vi "setROI.vi"(0 "PCO in":refnum<class "PCO_Camera.lvclass">, 7 "Seperator":string, 9 "value":string, 11 "error in (no error)":errorcluster) -> (4 "PCO out":refnum<class "PCO_Camera.lvclass">, 6 "output cluster":T1, 8 "value":dbl, 10 "Command out":string, 15 "error out":errorcluster)   [LabVIEW 2020, in "PCO_Camera.lvclass"]
uses:
  PCO_Camera.lvclass
  C:/GEECS/Developers Version/source/Device Drivers/Point Grey Camera/Point Grey Camera.lvclass
  ROI_TypDef.ctl
  PCO_Camera.lvclass/PCO_Camera.ctl
  Point Grey Camera.lvclass/Point Grey Camera.ctl
  Read Settings 2.vi
  Camera.lvclass
panel:
  out "ROI":u32[](array[numeric])
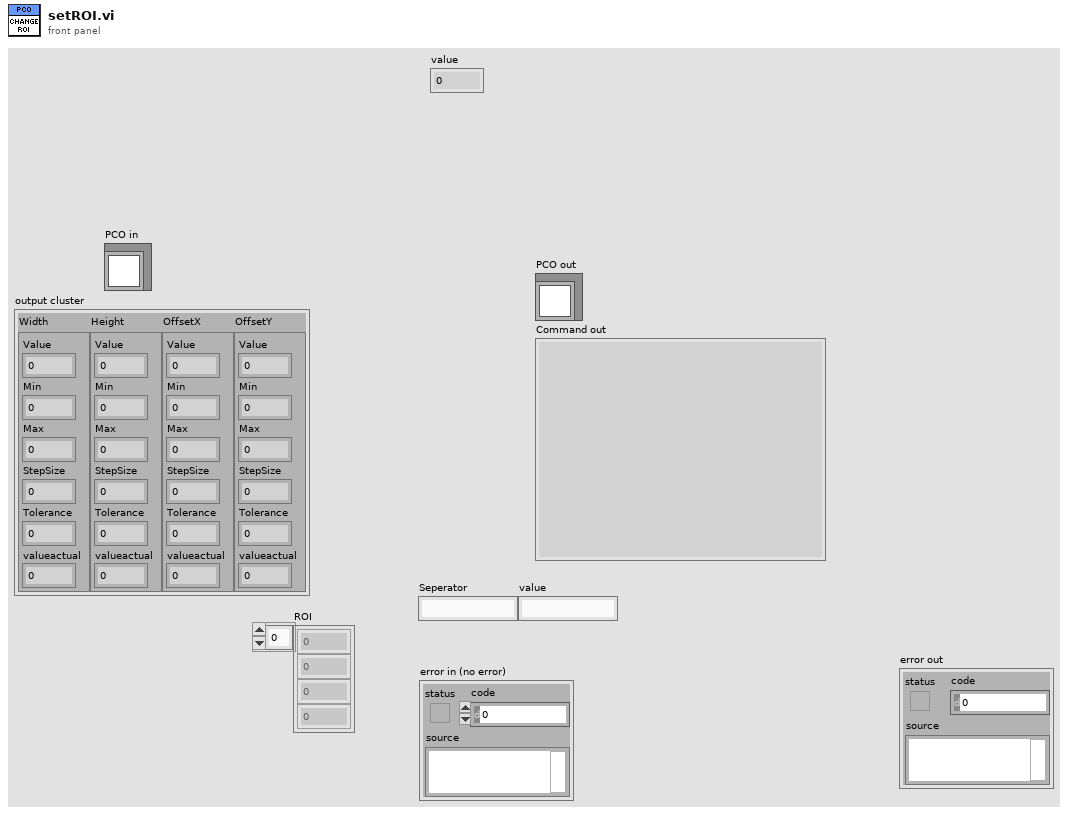
[diagram p1: front panel]
types:
  T1 = typedef "ROI_TypDef.ctl" = cluster{"Width":cluster{"Value":dbl, "Min":dbl, "Max":dbl, "StepSize":dbl, "Tolerance":dbl, "valueactual":dbl}, "Height":cluster{"Value":dbl, "Min":dbl, "Max":dbl, "StepSize":dbl, "Tolerance":dbl, "valueactual":dbl}, "OffsetX":cluster{"Value":dbl, "Min":dbl, "Max":dbl, "StepSize":dbl, "Tolerance":dbl, "valueactual":dbl}, "OffsetY":cluster{"Value":dbl, "Min":dbl, "Max":dbl, "StepSize":dbl, "Tolerance":dbl, "valueactual":dbl}}
  T2 = typedef "Point Grey Camera.lvclass/SettingsTypdef.ctl" = cluster{"Trigger":T3, "Gain":cluster{"Value":dbl, "Min":dbl, "Max":dbl, "StepSize":dbl, "Tolerance":dbl, "valueactual":dbl}, "Exposure":cluster{"Value":dbl, "Min":dbl, "Max":dbl, "StepSize":dbl, "Tolerance":dbl, "valueactual":dbl}, "Timeout":cluster{"Value":dbl, "Min":dbl, "Max":dbl, "StepSize":dbl, "Tolerance":dbl, "valueactual":dbl}, "LocalSavingPath":path, "Save":T3, "TriggerDelay":cluster{"Value":dbl, "Min":dbl, "Max":dbl, "StepSize":dbl, "Tolerance":dbl, "valueactual":dbl}, "CamSession":string, "ROI":T1, "MaxGUIPixel":cluster{"Value":dbl, "Min":dbl, "Max":dbl, "StepSize":dbl, "Tolerance":dbl, "valueactual":dbl}, "Target":cluster{"X":cluster{"Value":dbl, "Min":dbl, "Max":dbl, "StepSize":dbl, "Tolerance":dbl, "valueactual":dbl}, "Y":cluster{"Value":dbl, "Min":dbl, "Max":dbl, "StepSize":dbl, "Tolerance":dbl, "valueactual":dbl}}, "Analysis":T3, "maxshot#":dbl, "SpatialCalibration":cluster{"Value":dbl, "Min":dbl, "Max":dbl, "StepSize":dbl, "Tolerance":dbl, "valueactual":dbl}, "roistatus":T3, "Lineout":T3, "AnalysisThreshold":cluster{"Value":dbl, "Min":dbl, "Max":dbl, "StepSize":dbl, "Tolerance":dbl, "valueactual":dbl}, "TargetSize":cluster{"X":cluster{"Value":dbl, "Min":dbl, "Max":dbl, "StepSize":dbl, "Tolerance":dbl, "valueactual":dbl}, "Y":cluster{"Value":dbl, "Min":dbl, "Max":dbl, "StepSize":dbl, "Tolerance":dbl, "valueactual":dbl}}, "Simulation":T3, "SpatialCalibrationY":cluster{"Value":dbl, "Min":dbl, "Max":dbl, "StepSize":dbl, "Tolerance":dbl, "valueactual":dbl}, "Target2":cluster{"X":cluster{"Value":dbl, "Min":dbl, "Max":dbl, "StepSize":dbl, "Tolerance":dbl, "valueactual":dbl}, "Y":cluster{"Value":dbl, "Min":dbl, "Max":dbl, "StepSize":dbl, "Tolerance":dbl, "valueactual":dbl}}, "Target2Size":cluster{"X":cluster{"Value":dbl, "Min":dbl, "Max":dbl, "StepSize":dbl, "Tolerance":dbl, "valueactual":dbl}, "Y":cluster{"Value":dbl, "Min":dbl, "Max":dbl, "StepSize":dbl, "Tolerance":dbl, "valueactual":dbl}}, "Crosshair":cluster{"Label1":string, "Label2":string}, "Max2ndMomRadius":cluster{"Value":dbl, "Min":dbl, "Max":dbl, "StepSize":dbl, "Tolerance":dbl, "valueactual":dbl}, "SaveType":T4, "BackgroundPath":path, "GUI8bit":T3, "GUICompression":T3, "CompressionQuality":cluster{"Value":dbl, "Min":dbl, "Max":dbl, "StepSize":dbl, "Tolerance":dbl, "valueactual":dbl}, "SaveAsync":T3, "PerspectivePath":path, "PerspectiveCorrectGUI":T3, "BlackLevel":cluster{"Value":dbl, "Min":dbl, "Max":dbl, "StepSize":dbl, "Tolerance":dbl, "valueactual":dbl}, "TargetBP":cluster{"X":cluster{"Value":dbl, "Min":dbl, "Max":dbl, "StepSize":dbl, "Tolerance":dbl, "valueactual":dbl}, "Y":cluster{"Value":dbl, "Min":dbl, "Max":dbl, "StepSize":dbl, "Tolerance":dbl, "valueactual":dbl}}, "PythonAnalysis":T3, "PythonFunctionName":string, "PythonLineout":T3, "PythonVersion":string, "GEECSBuildsPath":path, "DisplayPythonProcessedImage":T3, "PythonModuleName":string, "AnalysisThresholdHigh":cluster{"Value":dbl, "Min":dbl, "Max":dbl, "StepSize":dbl, "Tolerance":dbl, "valueactual":dbl}, "AnalysisMedianRank":cluster{"Value":dbl, "Min":dbl, "Max":dbl, "StepSize":dbl, "Tolerance":dbl, "valueactual":dbl}, "ClockSpeed":cluster{"Value":dbl, "Min":dbl, "Max":dbl, "StepSize":dbl, "Tolerance":dbl, "valueactual":dbl}, "AutoTrigger":T3, "AutoTriggerLevelMeanCounts":cluster{"Value":dbl, "Min":dbl, "Max":dbl, "StepSize":dbl, "Tolerance":dbl, "valueactual":dbl}, "AnalysisROILeft":cluster{"Value":dbl, "Min":dbl, "Max":dbl, "StepSize":dbl, "Tolerance":dbl, "valueactual":dbl}, "AnalysisROIRight":cluster{"Value":dbl, "Min":dbl, "Max":dbl, "StepSize":dbl, "Tolerance":dbl, "valueactual":dbl}, "AnalysisROITop":cluster{"Value":dbl, "Min":dbl, "Max":dbl, "StepSize":dbl, "Tolerance":dbl, "valueactual":dbl}, "AnalysisROIBottom":cluster{"Value":dbl, "Min":dbl, "Max":dbl, "StepSize":dbl, "Tolerance":dbl, "valueactual":dbl}, "AnalysisROI":T3, "UseSoftwareTrigger":T3, "UDPtrigger":T3, "AutoTriggerLevelMaxCounts":cluster{"Value":dbl, "Min":dbl, "Max":dbl, "StepSize":dbl, "Tolerance":dbl, "valueactual":dbl}}
  T3 = typedef "OnOffTypeDef.ctl" = enum16{"off", "on"}
  T4 = typedef "Image save type.ctl" = enum16{"PNG", "BMP", "JPEG", "TDMS", "hdf5"}
  T5 = enum16{"sequence", "sequence non blocking", "ring buffer", "fifo", "sequence_dpcore", "sequence_non_blocking_dpcore", "ring_buffer_dpcore", "fifo_dpcore", "tif", "multitif", "pcoraw", "b16", "dicom", "multidicom"}
  T6 = typedef "Camera.lvclass/binning.ctl" = cluster{"vert":u16, "horz":u16}
  T7 = cluster{"exposure_time_s":dbl, "delay_time_s":dbl, "roi":cluster{"x0":u64, "y0":u64, "x1":u64, "y1":u64}, "timestamp_mode":u16, "pixelrate":u32, "trigger_mode":u16, "acquire_mode":u16, "metadata_mode":u16, "noisefilter_mode":u16, "binning":T6}
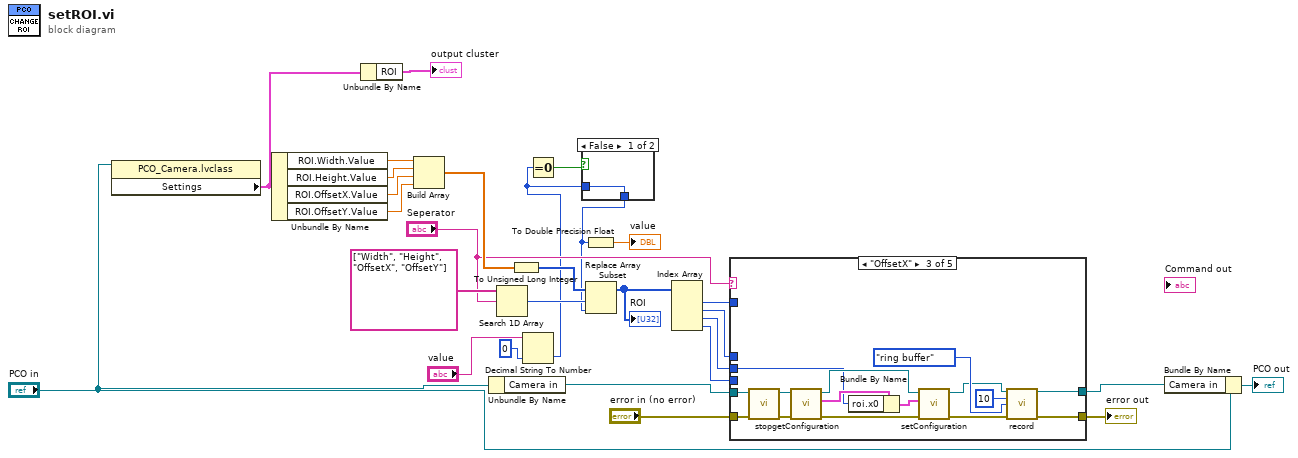
[diagram p0: block diagram]
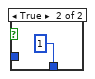
[diagram p2: hidden frame]
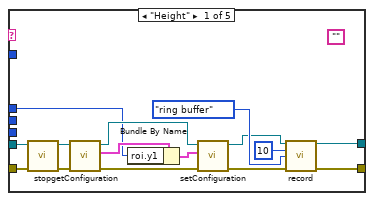
[diagram p3: hidden frame]
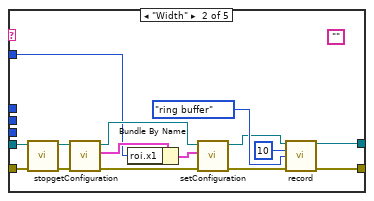
[diagram p4: hidden frame]
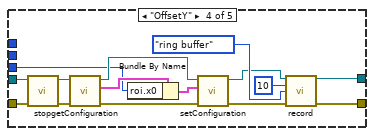
[diagram p5: hidden frame]
diagram:
  n1 = property class="PCO_Camera.lvclass"(reference="PCO in") -> ("Settings"=w5:T2)  [unwired: 1 in, 2 out]
  n2 = Unbundle By Name(w5) -> ("ROI.Width.Value"=w23:dbl, "ROI.Height.Value"=w22:dbl, "ROI.OffsetX.Value"=w21:dbl, "ROI.OffsetY.Value"=w20:dbl)
  n3 = Unbundle By Name(w5) -> ("ROI"=→"output cluster":T1)
  n4 = Build Array(w23, w22, w21, w20) -> (w19:dbl[])
  n5 = Unbundle By Name("PCO in") -> ("Camera in"=w15:refnum<class "Camera.lvclass">)
  n6 = Search 1D Array(1D array=string[] ["Width", "Height", "OffsetX", "OffsetY"] ("Seperator"), element="Seperator") -> (index of element=w25:i32)  [unwired: 1 in]
  n7 = To Unsigned Long Integer(number=w19) -> (unsigned 32bit integer=w26:u32[])
  n8 = Decimal String To Number(string="value", default (0L)=u32 0 ("default (0 I32)")) -> (number=w2:u32)  [unwired: 1 in, 1 out]
  n9 = Equal To 0?(x=w2) -> (x = 0?=w3:bool)
  n10 = case shown="False" w3 {
    tunnel: [w29 1] -> w1
    tunnel: w2 -> [w29 _]
    frame False {
    }
    frame True {
    }
  }
  n11 = To Double Precision Float(number=w1) -> (double precision float=→"value":dbl)
  n12 = Replace Array Subset(array=w26, new element=w1, index=w25) -> (w24:u32[])
  "ROI" <- w24
  n13 = Index Array(array=w24) -> (element #1=w14:u32, element #2=w13:u32, element #3=w12:u32, element #4=w11:u32)  [unwired: 4 in]
  n14 = case shown="\"OffsetX\"" "Seperator" {
    tunnel: w15 -> [w39 w54 w69 w84 w92]
    tunnel: [w36 w51 w66 w81 w92] -> w10
    tunnel: w14 -> [_ w48 _ _ _]
    tunnel: w13 -> [w33 _ _ _ _]
    tunnel: w12 -> [_ _ w63 _ _]
    tunnel: w11 -> [_ _ _ w78 _]
    tunnel: "error in (no error)" -> [w32 w47 w62 w77 w91]
    tunnel: [w31 w46 w61 w76 w91] -> w6
    frame "Height" {
      (unwired) ""
      n15 = call-dynamic "stop.vi"("error in (no error)"=w32, "Camera in"=w39) -> ("error out"=w44:errorcluster, "Camera out"=w43:refnum<class "Camera.lvclass">)  [unwired: 8 in]
      n16 = call-dynamic "getConfiguration.vi"("error in (no error)"=w44, "Camera in"=w43) -> ("error out"=w42:errorcluster, "configuration"=w34:T7, "Camera out"=w38:refnum<class "Camera.lvclass">)  [unwired: 7 in]
      n17 = Bundle By Name(cluster=w34, "roi.y1"=w33) -> (w35:T7)
      n18 = call-dynamic "setConfiguration.vi"("error in (no error)"=w42, "configuration"=w35, "Camera in"=w38) -> ("error out"=w45:errorcluster, "Camera out"=w37:refnum<class "Camera.lvclass">)  [unwired: 7 in]
      n19 = call-dynamic "record.vi"("Camera in"=w37, "num_images"=u32 10, "record_mode"=T5."ring buffer", "error in (no error)"=w45) -> ("Camera out"=w36:refnum<class "Camera.lvclass">, "error out"=w31:errorcluster)  [unwired: 10 in]
    }
    frame "Width" {
      (unwired) ""
      n20 = call-dynamic "stop.vi"("error in (no error)"=w47, "Camera in"=w54) -> ("error out"=w59:errorcluster, "Camera out"=w58:refnum<class "Camera.lvclass">)  [unwired: 8 in]
      n21 = call-dynamic "getConfiguration.vi"("error in (no error)"=w59, "Camera in"=w58) -> ("error out"=w57:errorcluster, "configuration"=w49:T7, "Camera out"=w53:refnum<class "Camera.lvclass">)  [unwired: 7 in]
      n22 = Bundle By Name(cluster=w49, "roi.x1"=w48) -> (w50:T7)
      n23 = call-dynamic "setConfiguration.vi"("error in (no error)"=w57, "configuration"=w50, "Camera in"=w53) -> ("error out"=w60:errorcluster, "Camera out"=w52:refnum<class "Camera.lvclass">)  [unwired: 7 in]
      n24 = call-dynamic "record.vi"("Camera in"=w52, "num_images"=u32 10, "record_mode"=T5."ring buffer", "error in (no error)"=w60) -> ("Camera out"=w51:refnum<class "Camera.lvclass">, "error out"=w46:errorcluster)  [unwired: 10 in]
    }
    frame "OffsetX" {
      n25 = call-dynamic "stop.vi"("error in (no error)"=w62, "Camera in"=w69) -> ("error out"=w74:errorcluster, "Camera out"=w73:refnum<class "Camera.lvclass">)  [unwired: 8 in]
      n26 = call-dynamic "getConfiguration.vi"("error in (no error)"=w74, "Camera in"=w73) -> ("error out"=w72:errorcluster, "configuration"=w64:T7, "Camera out"=w68:refnum<class "Camera.lvclass">)  [unwired: 7 in]
      n27 = Bundle By Name(cluster=w64, "roi.x0"=w63) -> (w65:T7)
      n28 = call-dynamic "setConfiguration.vi"("error in (no error)"=w72, "configuration"=w65, "Camera in"=w68) -> ("error out"=w75:errorcluster, "Camera out"=w67:refnum<class "Camera.lvclass">)  [unwired: 7 in]
      n29 = call-dynamic "record.vi"("Camera in"=w67, "num_images"=u32 10, "record_mode"=T5."ring buffer", "error in (no error)"=w75) -> ("Camera out"=w66:refnum<class "Camera.lvclass">, "error out"=w61:errorcluster)  [unwired: 10 in]
    }
    frame "OffsetY" {
      n30 = call-dynamic "stop.vi"("error in (no error)"=w77, "Camera in"=w84) -> ("error out"=w89:errorcluster, "Camera out"=w88:refnum<class "Camera.lvclass">)  [unwired: 8 in]
      n31 = call-dynamic "getConfiguration.vi"("error in (no error)"=w89, "Camera in"=w88) -> ("error out"=w87:errorcluster, "configuration"=w79:T7, "Camera out"=w83:refnum<class "Camera.lvclass">)  [unwired: 7 in]
      n32 = Bundle By Name(cluster=w79, "roi.x0"=w78) -> (w80:T7)
      n33 = call-dynamic "setConfiguration.vi"("error in (no error)"=w87, "configuration"=w80, "Camera in"=w83) -> ("error out"=w90:errorcluster, "Camera out"=w82:refnum<class "Camera.lvclass">)  [unwired: 7 in]
      n34 = call-dynamic "record.vi"("Camera in"=w82, "num_images"=u32 10, "record_mode"=T5."ring buffer", "error in (no error)"=w90) -> ("Camera out"=w81:refnum<class "Camera.lvclass">, "error out"=w76:errorcluster)  [unwired: 10 in]
    }
    frame "False", Default {
    }
  }
  "error out" <- w6
  n35 = Bundle By Name(cluster="PCO in", "Camera in"=w10) -> (→"PCO out":refnum<class "PCO_Camera.lvclass">)
